vi "Check If Valid.vi"(8 "error in (no error)":errorcluster, 11 "Messenger - Actor in":refnum<class "Messenger.lvclass">) -> (0 "error out":errorcluster, 2 "Is Valid":bool, 3 "Messenger - Actor out":refnum<class "Messenger.lvclass">)   [LabVIEW 2015, in "Messenger.lvclass"]
uses:
  Messenger.lvclass
  Messenger.lvclass/Messenger.ctl
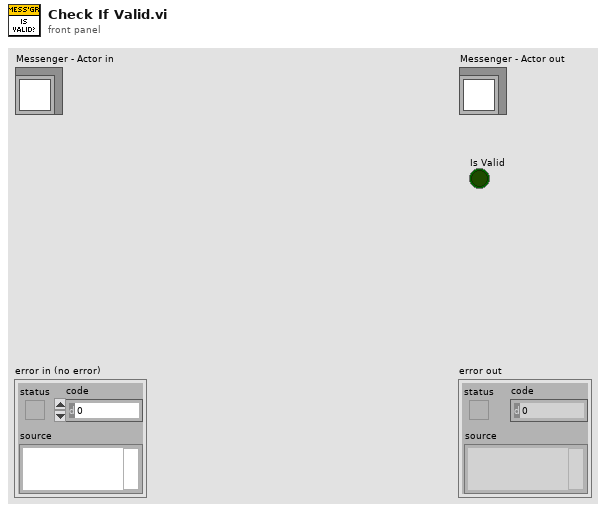
[diagram p1: front panel]
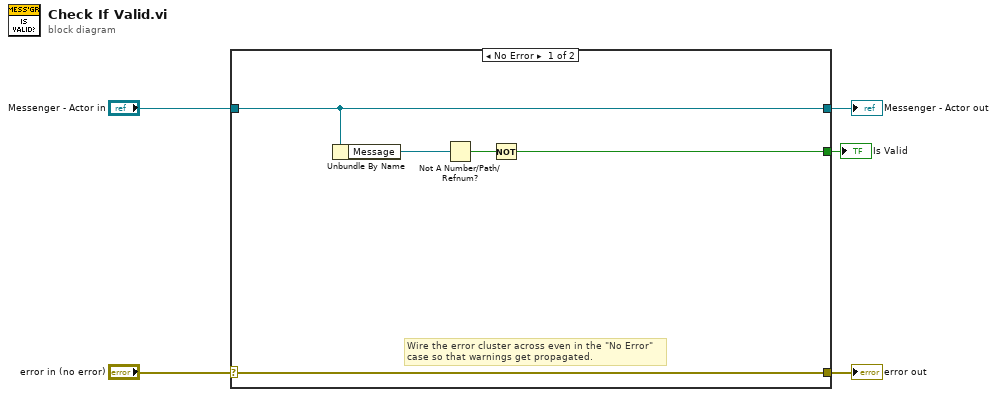
[diagram p0: block diagram]
diagram:
  n1 = case shown="No Error" "error in (no error)" {
    selector: "error in (no error)" -> [w10 w12]
    tunnel: [w10 w12] -> w4
    tunnel: [w9 w11] -> w2
    tunnel: "Messenger - Actor in" -> [w9 w11]
    tunnel: [w6 _] -> w1
    frame No Error {
      # "Wire the error cluster across even in the \"No Error\"\ncase so that warnings get propagated."
      n2 = Unbundle By Name(w9) -> ("Message"=w8:refnum<user-event>)
      n3 = Not A Number/Path/Refnum?(number/path/refnum=w8) -> (NaN/Path/Refnum?=w7:bool)
      n4 = Not(x=w7) -> (.not. x?=w6:bool)
    }
    frame Error {
    }
  }
  "error out" <- w4
  "Messenger - Actor out" <- w2
  "Is Valid" <- w1
